vi "Attributes.vi"() -> ()   [LabVIEW 2017]
panel:
  in  "attributes":string[](array[string])=["ID", "owner path", "display name", "parsable"]
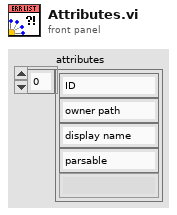
[diagram p1: front panel]
diagram:
